vi "Centrid.vi"() -> ()   [LabVIEW 2014]
doc: "Use this template to build a VI to use as a subVI."
uses:
  <vilib>/vision/NI_Vision_Development_Module.lvlib
panel:
  out "Centroid":cluster{"X Centroid":sgl, "Y Centroid":sgl} {"Y Centroid" format="%.2f"; "X Centroid" format="%.2f"}
  out "Src":T1(plugin-control)
  out "Centroid":T1(plugin-control)
  # ":: MVi Framework V1.0 ::\nAuthor:Gaoke Yang\nEmail: gaoke.yang@yahoo.com\nWeb: www.mvicontrol.com\nCopyright (C) 2015, MVI Technologies All Rights Reserved"
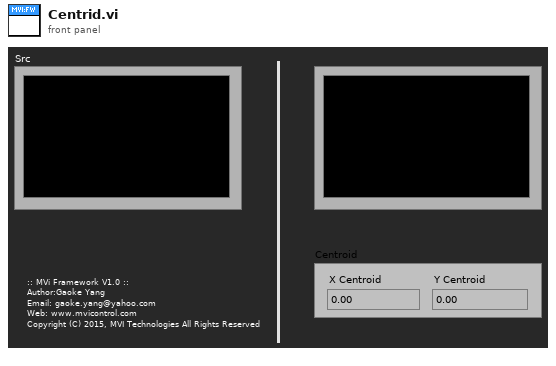
[diagram p1: front panel]
types:
  T1 = typedef "IMAQ Image.ctl" = refnum<image>
  T2 = cluster{"X Size":i32, "Y Size":i32, "% Tolerance":i32}
  T3 = typedef "Image Type" = u32
  T4 = typedef "ROI Descriptor" = cluster{"Global Rectangle":i32[], "Contours":cluster{"ID":enum32{"External", "Internal"}, "Type":u32, "Coordinates":i32[]}[]}
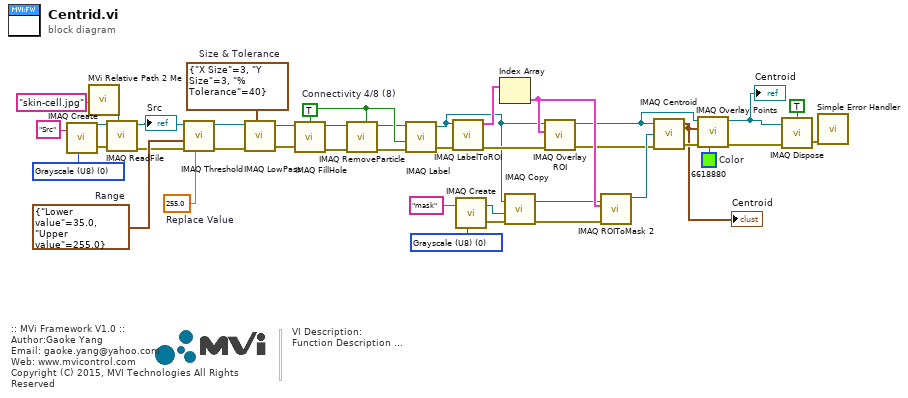
[diagram p0: block diagram]
diagram:
  w10 = TRUE  # Connectivity 4/8 (8)
  w11 = T2 {"X Size"=3, "Y Size"=3, "% Tolerance"=40}  # Size & Tolerance
  w15 = u32 6618880  # Color
  w17 = T3 0 items=["Grayscale (U8)", "Grayscale (I16)", "Grayscale (SGL)", "Complex (CSG)", "RGB (U32)", "HSL (U32)", "RGB (U64)", "Grayscale (U16)"] ("Image Type")
  w33 = cluster{"Lower value":sgl, "Upper value":sgl} {"Lower value"=35.0, "Upper value"=255.0}  # Range
  w28 = sgl 255.0  # Replace Value
  w35 = T3 0 items=["Grayscale (U8)", "Grayscale (I16)", "Grayscale (SGL)", "Complex (CSG)", "RGB (U32)", "HSL (U32)", "RGB (U64)", "Grayscale (U16)"] ("Image Type")
  # "VI Description:\nFunction Description ..."
  # ":: MVi Framework V1.0 ::\nAuthor:Gaoke Yang\nEmail: gaoke.yang@yahoo.com\nWeb: www.mvicontrol.com\nCopyright (C) 2015, MVI Technologies All Rights Reserved"
  n1 = call "IMAQ Create"("Image Name"="Src" ("name or relative path"), "Image Type"=w35) -> ("New Image"=w36:T1, "error out"=w34:errorcluster)  [unwired: 2 in, 1 out]
  n2 = call "MVi Relative Path 2 Me.vi"("Relative Path"="skin-cell.jpg" ("name or relative path")) -> ("Appended Dir"=w37:path)  [unwired: 5 in, 1 out]
  n3 = call "IMAQ ReadFile"("File Path"=w37, "error in (no error)"=w34, "Image"=w36) -> ("error out"=w32:errorcluster, "Image Out"=w12:T1)  [unwired: 4 in, 3 out]
  "Src" <- w12
  n4 = call "IMAQ Threshold"("Replace Value"=w28, "error in (no error)"=w32, "Range"=w33, "Image Src"=w12) -> ("error out"=w31:errorcluster, "Image Dst Out"=w29:T1)  [unwired: 6 in]
  n5 = call "IMAQ LowPass"("Image Src"=w29, "Size & Tolerance"=w11, "error in (no error)"=w31) -> ("Image Dst Out"=w2:T1, "error out"=w30:errorcluster)  [unwired: 4 in]
  n6 = call "IMAQ FillHole"("error in (no error)"=w30, "Image Src"=w2, "Connectivity 4/8 (8)"=w10) -> ("error out"=w27:errorcluster, "Image Dst Out"=w3:T1)  [unwired: 3 in]
  n7 = call "IMAQ RemoveParticle"("Connectivity 4/8 (8)"=w10, "error in (no error)"=w27, "Image Src"=w3) -> ("error out"=w26:errorcluster, "Image Dst Out"=w4:T1)  [unwired: 7 in]
  n8 = call "IMAQ Label"("error in (no error)"=w26, "Connectivity 4/8 (8)"=w10, "Image Src"=w4) -> ("error out"=w25:errorcluster, "Image Dst Out"=w5:T1)  [unwired: 1 in, 1 out]
  n9 = call "IMAQ LabelToROI"("error in (no error)"=w25, "Image"=w5) -> ("error out"=w9:errorcluster, "ROIs"=w24:T4[])  [unwired: 6 in, 2 out]
  n10 = call "IMAQ Create"("Image Name"="mask" ("name or relative path"), "Image Type"=w17) -> ("New Image"=w14:T1, "error out"=w13:errorcluster)  [unwired: 2 in, 1 out]
  n11 = Index Array(array=w24) -> (element=w23:T4)  [unwired: 1 in]
  n12 = call "IMAQ Copy"("error in (no error)"=w13, "Image Dst"=w14, "Image Src"=w5) -> ("error out"=w7:errorcluster, "Image Dst Out"=w8:T1)  [unwired: 3 in]
  n13 = call "IMAQ Overlay ROI"("error in (no error)"=w9, "ROI Descriptor"=w23, "Image"=w5) -> ("error out"=w6:errorcluster, "Image Out"=w19:T1)  [unwired: 7 in]
  n14 = call "IMAQ ROIToMask 2"("error in (no error)"=w7, "ROI Descriptor"=w23, "Image"=w8) -> ("Image Out"=w22:T1)  [unwired: 6 in, 2 out]
  n15 = call "IMAQ Centroid"("error in (no error)"=w6, "Image Mask"=w22, "Image"=w19) -> ("error out"=w21:errorcluster, "Centroid"=w18:cluster{"X Centroid":sgl, "Y Centroid":sgl})  [unwired: 1 in]
  "Centroid" <- w18
  n16 = call "IMAQ Overlay Points"("Color"=w15, "error in (no error)"=w21, "Point"=w18, "Image"=w19) -> ("error out"=w20:errorcluster, "Image Out"=w1:T1)  [unwired: 6 in]
  "Centroid" <- w1
  n17 = call "IMAQ Dispose"("All Images? (No)"=TRUE, "Image"=w1, "error in (no error)"=w20) -> ("error out"=w38:errorcluster)  [unwired: 3 out]
  n18 = call <vilib>:"Simple Error Handler.vi"("error in (no error)"=w38) -> ()  [unwired: 1 in, 8 out]
